vi "Number-to-hex-2-digit.vi"(11 "dec_num":i32) -> (3 "hex_num":string)   [LabVIEW 2014]
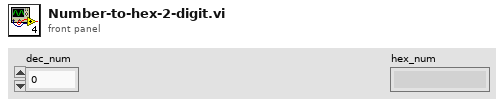
[diagram p1: front panel]
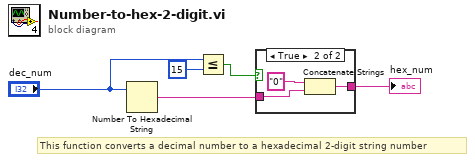
[diagram p0: block diagram]
diagram:
  # "This function converts a decimal number to a hexadecimal 2-digit string number"
  n1 = Number To Hexadecimal String(2:"dec_num") -> (0:w5:string)  [unwired: 1 in]
  n2 = Less Or Equal?(x="dec_num", y=15) -> (x <= y?=w4:bool)
  n3 = case shown="True" w4 {
    tunnel: [w6 w9] -> w1
    tunnel: w5 -> [w6 w7]
    frame False {
    }
    frame True {
      n4 = Concatenate Strings("0" ("string"), w7) -> (w9:string)
    }
  }
  "hex_num" <- w1
